vi "Add Peça.vi"(0 "Limite Vertical":sgl, 1 "X médio":sgl, 2 "Y médio":sgl, 3 "Array Cluster in":T1(array[cluster]), 4 "Dados":string) -> (5 "Array Cluster out":T1(array[cluster]))   [LabVIEW 2020]
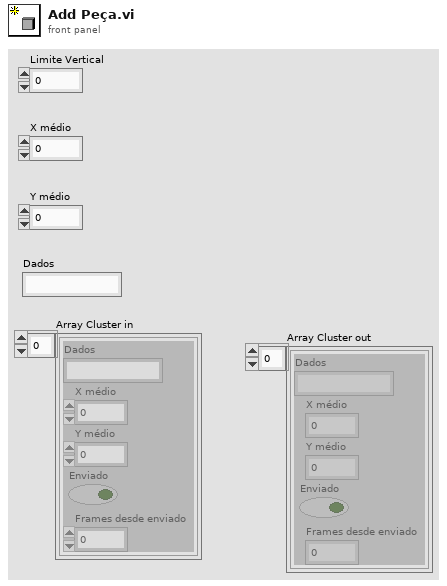
[diagram p1: front panel]
types:
  T1 = cluster{"Dados":string, "X médio":dbl, "Y médio":dbl, "Enviado":bool, "Frames desde enviado":dbl}[]
  T2 = cluster{"Dados":string, "X médio":dbl, "Y médio":dbl, "Enviado":bool, "Frames desde enviado":dbl}
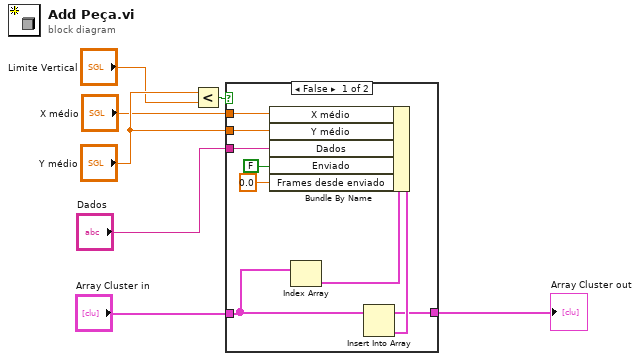
[diagram p0: block diagram]
diagram:
  n1 = Less?(x="Y médio", y="Limite Vertical") -> (x < y?=w4:bool)
  n2 = case shown="False" w4 {
    tunnel: "X médio" -> [w16 _]
    tunnel: "Y médio" -> [w15 _]
    tunnel: "Dados" -> [w14 _]
    tunnel: "Array Cluster in" -> [w10 w17]
    tunnel: [w8 w17] -> w7
    frame False {
      n3 = Index Array(array=w10) -> (element=w11:T2)  [unwired: 1 in]
      n4 = Bundle By Name(cluster=w11, "X médio"=w16, "Y médio"=w15, "Dados"=w14, "Enviado"=FALSE, "Frames desde enviado"=0.0 ("Frames sem atualização")) -> (w9:T2)
      n5 = Insert Into Array(array=w10, new element=w9) -> (w8:T1)  [unwired: 1 in]
    }
    frame True {
    }
  }
  "Array Cluster out" <- w7
